vi "Stop Core.vi"(10 "final error code":i32, 11 "ReceiverState in":refnum<class "Connect Command.lvclass">) -> (3 "ReceiverState out":refnum<class "Connect Command.lvclass">)   [LabVIEW 2013, in "Receiver.lvlib" / "Commands.lvlib" / "Connect.lvlib" / "Connect Command.lvclass"]
doc: "(<B>Filename</B>: Actor Framework.lvlib:Actor.lvclass:Stop Core.vi)\n\nDefines what the actor does before it stops. Use the <B>final error code</B> input to determine whether the actor shut down in response to an error.\n\nBy default, this method does nothing. A descendant class may override it to define behavior, such as shutting down any processes the actor initiated in its override of the Actor Core method."
uses:
  Connect Command.lvclass
  Receiver Commands/Command Processor.lvclass
  Connect Command.lvclass/Connect Command.ctl
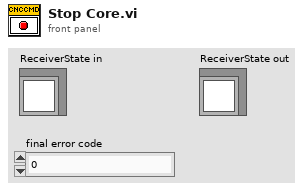
[diagram p1: front panel]
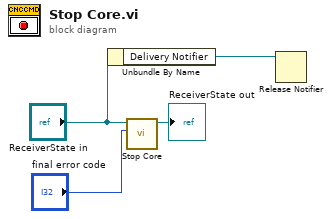
[diagram p0: block diagram]
diagram:
  n1 = Unbundle By Name("ReceiverState in") -> ("Delivery Notifier"=w1:refnum<notifier>)
  n2 = call-parent "Stop Core.vi"("final error code"="final error code", "Command Processor in"="ReceiverState in") -> ("Command Processor out"=→"ReceiverState out":refnum<class "Connect Command.lvclass">)  [unwired: 9 in]
  n3 = Release Notifier(notifier=w1) -> ()  [unwired: 2 in, 3 out]
